vi "lsl create inlet.vi"(7 "recover":i32, 8 "error in (no error)":errorcluster, 9 "max_chunklen":i32, 10 "max_buflen":i32, 11 "info":cluster{}) -> (0 "error out":errorcluster, 2 "function return":u32, 3 "info out":cluster{})   [LabVIEW 2018, in "liblsl-LabVIEW.lvlib"]
doc: "extern LIBLSL_C_API lsl_inlet lsl_create_inlet(lsl_streaminfo info, int32_t max_buflen, int32_t max_chunklen, int32_t recover);"
uses:
  <userlib>/liblsl-LabVIEW/liblsl-LabVIEW.lvlib
  <userlib>/liblsl-LabVIEW/liblsl64.dll
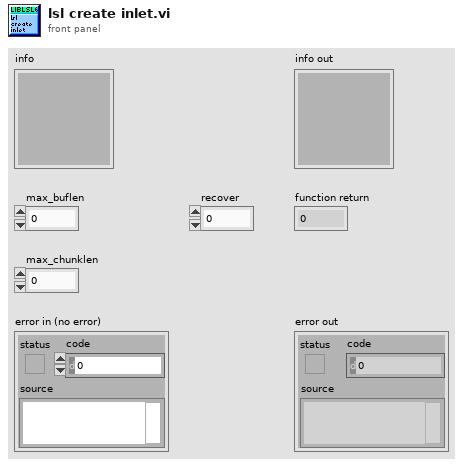
[diagram p1: front panel]
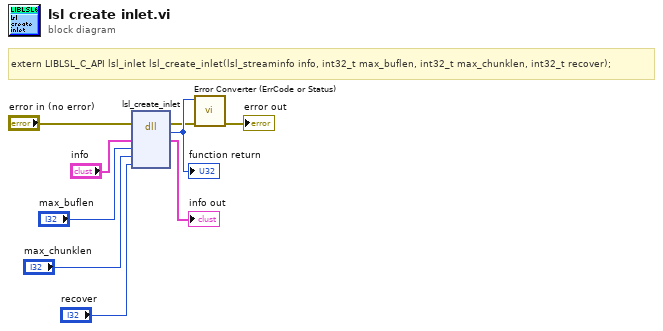
[diagram p0: block diagram]
diagram:
  # "extern LIBLSL_C_API lsl_inlet lsl_create_inlet(lsl_streaminfo info, int32_t max_buflen, int32_t max_chunklen, int32_t recover);"
  n1 = dll-call lib="C:/Program Files/National Instruments/LabVIEW 2018/user.lib/liblsl-LabVIEW/liblsl64.*" fn="lsl_create_inlet"(error in="error in (no error)", "info"="info", "max_buflen"="max_buflen", "max_chunklen"="max_chunklen", "recover"="recover") -> (error out=w2:errorcluster, w9:u32, "info"=→"info out":cluster{})  [unwired: 5 in, 1 out]
  "function return" <- w9
  n2 = call <userlib>:"Error Converter (ErrCode or Status).vi"("error in (no error)"=w2, "error code"=w9) -> ("error out"=→"error out":errorcluster)  [unwired: 9 in]
